vi "S2C_CMD_LoadCmds.vi"(8 "Error In":errorcluster, 11 "Driver":string) -> (0 "Error Out":errorcluster)   [LabVIEW 2015]
doc: "Performs a function lookup on the 4D arrays and load the values into the Command and Type active arrays."
uses:
  S2C_CMD_Globals.vi
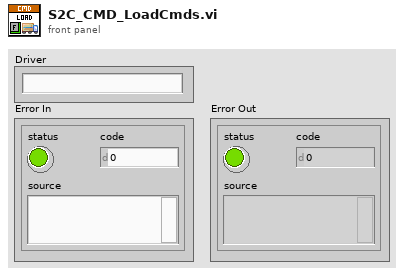
[diagram p1: front panel]
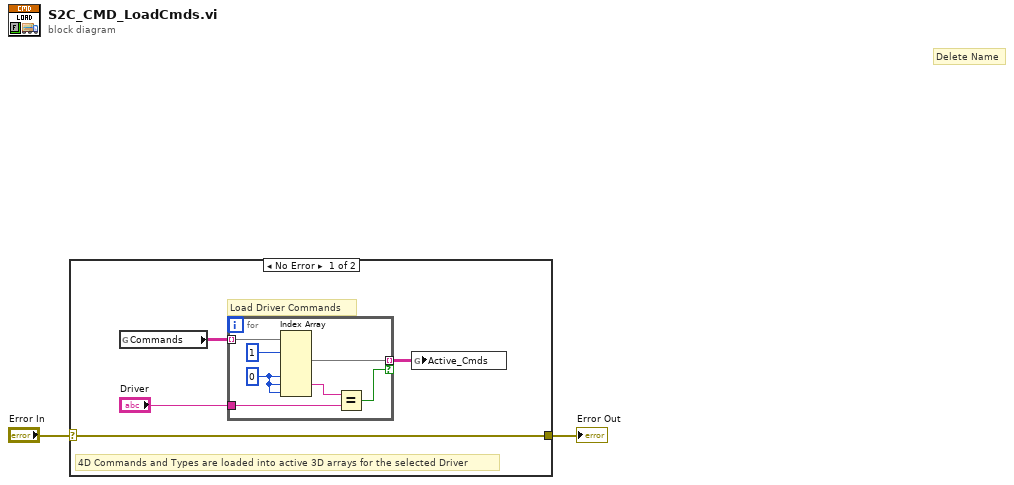
[diagram p0: block diagram]
diagram:
  # "Delete Name"
  n1 = case shown="No Error" "Error In" {
    selector: "Error In" -> [w6 w14]
    tunnel: [w6 w14] -> w1
    frame No Error {
      # "4D Commands and Types are loaded into active 3D arrays for the selected Driver"
      # "Load Driver Commands"
      n2 = global read "S2C_CMD_Globals.vi" "Commands"() -> (w5:string[][][][])
      n3 = for {
        tunnel: w5 -> [w13] mode=indexing
        tunnel: "Driver" -> [w12]
        tunnel: [w9] -> w4 mode=indexing if=w8
        w11 = 0 ("index (page)")
        n4 = Index Array(array=w13, index (dim 0) #1=1 ("index (page)"), index (dim 0) #2=w11, index (dim 1) #2=w11, index (dim 2) #2=w11) -> (element #1=w9:string[][], element #2=w10:string)  [unwired: 2 in]
        n5 = Equal?(x=w10, y=w12) -> (x = y?=w8:bool)
      }
      n6 = global write "S2C_CMD_Globals.vi" "Active_Cmds"(w4) -> ()
    }
    frame Error {
    }
  }
  "Error Out" <- w1
